vi "InsertStringCorrection.vi"(4 "SQL string":string) -> (1 "SQL String Out":string)   [LabVIEW 2020, in "ORM_DBC_Npgsql.lvlib" / "DBC.lvclass"]
doc: "With postgreSQL, table and column names must be lower case. The default column names for the \"Log\" table are hardwired in Log Action.vi as mixed case. This VI looks for the default column names and changes them to all lower case. If all the expected column names are not found, the input string is passed through to the output unchanged."
uses:
  DBC.lvclass
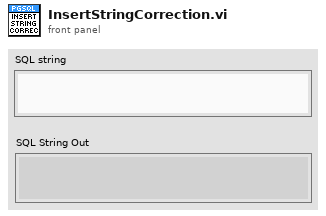
[diagram p1: front panel]
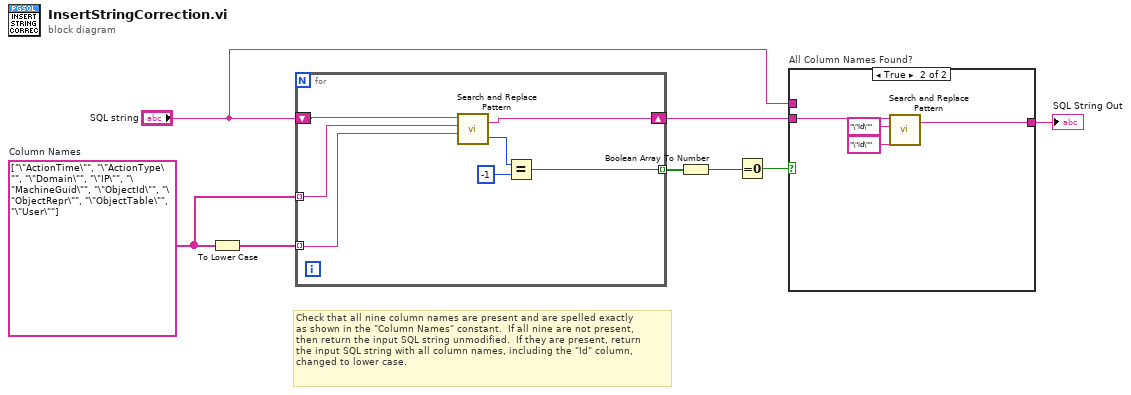
[diagram p0: block diagram]
diagram:
  w7 = string[] ["\"ActionTime\"", "\"ActionType\"", "\"Domain\"", "\"IP\"", "\"MachineGuid\"", "\"ObjectId\"", "\"ObjectRepr\"", "\"ObjectTable\"", "\"User\""]  # Column Names
  # "Check that all nine column names are present and are spelled exactly\nas shown in the \"Column Names\" constant.  If all nine are not present,\nthen return the input SQL string unmodified.  If they are present, return\nthe input SQL string with all column names, including the \"Id\" column,\nchanged to lower case."
  n1 = To Lower Case(string=w7) -> (all lower case string=w8:string[])
  n2 = for {
    shift-right: [w9] -> w3
    shift-left: "SQL string" -> [w15]
    tunnel: w8 -> [w13] mode=indexing
    tunnel: w7 -> [w14] mode=indexing
    tunnel: [w10] -> w6 mode=indexing
    n3 = call <vilib>:"Search and Replace Pattern.vi"("string"=w15, "regular expression (\"\")"=w14, "replace string (\"\")"=w13) -> ("result string"=w9:string, "offset past match"=w12:i32)  [unwired: 2 in]
    n4 = Equal?(x=w12, y=-1) -> (x = y?=w10:bool)
  }
  n5 = Boolean Array To Number(Boolean array=w6) -> (number=w5:u32)
  n6 = Equal To 0?(x=w5) -> (x = 0?=w4:bool)
  n7 = case "All Column Names Found?" shown="True" w4 {
    tunnel: w3 -> [_ w20]
    tunnel: "SQL string" -> [w16 _]
    tunnel: [w16 w17] -> w1
    frame False {
    }
    frame True {
      n8 = call <vilib>:"Search and Replace Pattern.vi"("string"=w20, "regular expression (\"\")"="\"Id\"" ("regular expression (\"\")"), "replace string (\"\")"="\"id\"" ("replace string (\"\")")) -> ("result string"=w17:string)  [unwired: 2 in, 1 out]
    }
  }
  "SQL String Out" <- w1
